vi "LD settings.vi"(8 "Error In":errorcluster, 10 "General information in":T1 {"LD ID" min=0 max=1000 step=1}, 11 "mode (R)":enum16{"read", "write"}(ring)) -> (0 "Error out":errorcluster, 2 "general information out":T1 {"LD ID" min=0 max=1000 step=1})   [LabVIEW 2014]
doc: "Functional Global Variable for the algorithm settings. The used method as well as the max. Iteration steps and the tolerance can be given. In addition, the algorithm can be told to use boundaries (if possible)."
uses:
  controls/LD settings.ctl
panel:
  # "Input"
  # "Output"
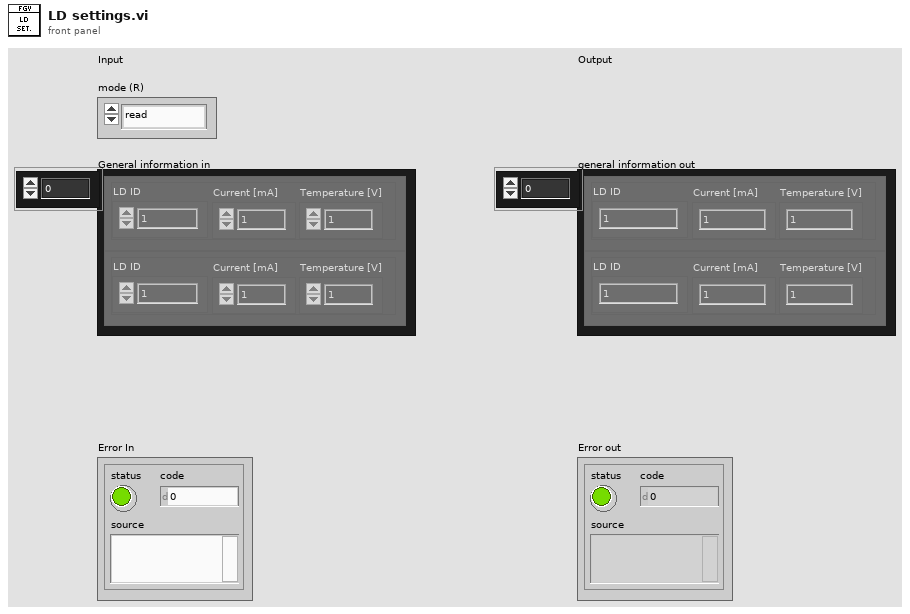
[diagram p1: front panel]
types:
  T1 = typedef "LD settings.ctl" = cluster{"LD ID":i32, "Current [mA]":dbl, "Temperature [V]":dbl}[]
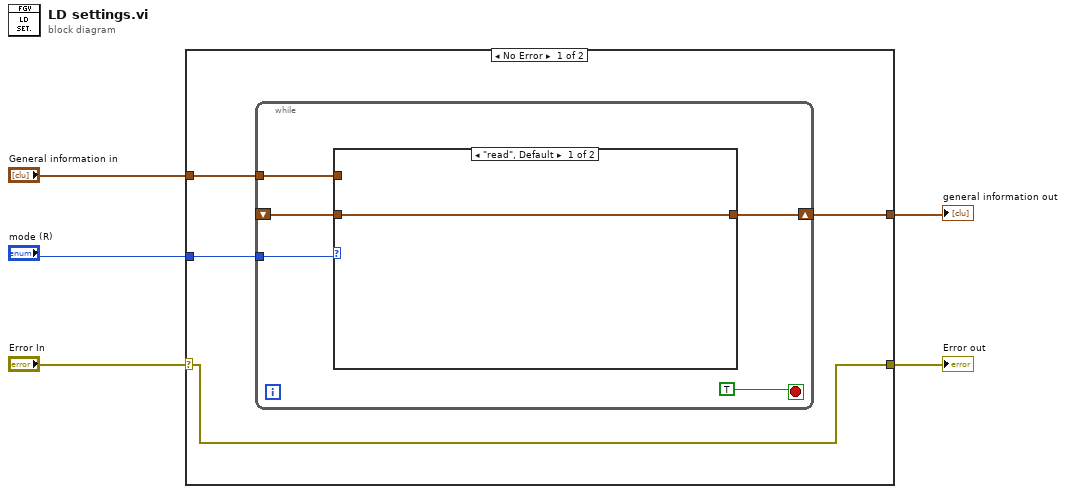
[diagram p0: block diagram]
diagram:
  n1 = case shown="No Error" "Error In" {
    selector: "Error In" -> [w6 w18]
    tunnel: "mode (R)" -> [w9 _]
    tunnel: [w6 w18] -> w4
    tunnel: "General information in" -> [w8 w17]
    tunnel: [w7 w17] -> w2
    frame No Error {
      n2 = while {
        tunnel: w9 -> [w13]
        tunnel: w8 -> [w12]
        shift-right: [w10] -> w7
        shift-left: _ -> [w11]
        stop <- TRUE stop-if-true
        n3 = case shown="\"read\", Default" w13 {
          tunnel: w12 -> [_ w16]
          tunnel: w11 -> [w15 _]
          tunnel: [w15 w16] -> w10
          frame "read", Default {
          }
          frame "write" {
          }
        }
      }
    }
    frame Error {
    }
  }
  "Error out" <- w4
  "general information out" <- w2
